vi "Delete Active DUT SIM Slot.vi"(8 "error in (no error)":errorcluster, 10 "SIM Slot (1)":i32=1, 11 "VISA resource name":refnum<visa-resource-name>) -> (0 "error out":errorcluster, 3 "VISA resource name out":refnum<visa-resource-name>)   [LabVIEW 2015, in "Rohde&Schwarz CMXP Base.lvlib"]
doc: "Removes the SIM slot with the number from the active DUT.\n\nAttribute:\nRSCMXPBASE_ATTR_ACTIVE_DUT_SIM_SLOT_DELETE\n\nRemote-control command:\nDELete:DUT:SIMSlot"
uses:
  <instrlib>/Rohde&Schwarz CMXP Base/Rohde&Schwarz CMXP Base.lvlib
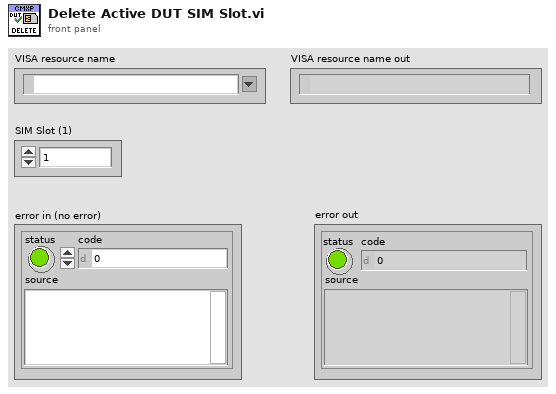
[diagram p1: front panel]
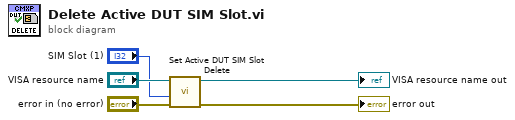
[diagram p0: block diagram]
diagram:
  n1 = call "Set Active DUT SIM Slot Delete"("error in (no error)"="error in (no error)", "Active DUT SIM Slot Delete (0)"="SIM Slot (1)", "instrument handle"="VISA resource name") -> ("error out"=→"error out":errorcluster, "instrument handle out"=→"VISA resource name out":refnum<visa-resource-name>)  [unwired: 7 in]
